vi "SecondsToHMS.vi"() -> ()   [LabVIEW 2014]
panel:
  out "Seconds":dbl
  out "Minutes":dbl
  out "Hours":dbl
  in  "Total Time in Seconds":dbl
  # "Converts time in seconds to hours, minutes and seconds"
  # "Control"
  # "Indicator"
  # "Indicator"
  # "Indicator"
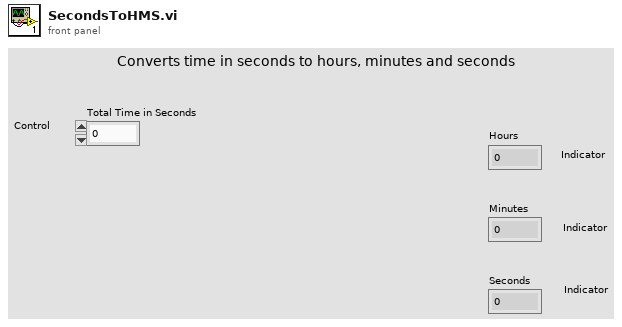
[diagram p1: front panel]
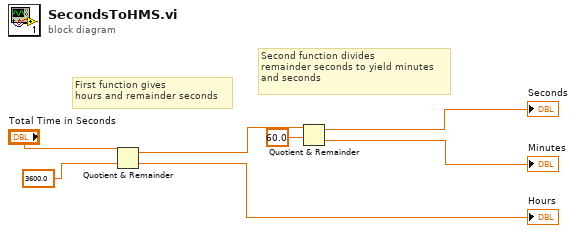
[diagram p0: block diagram]
diagram:
  # "Second function divides\nremainder seconds to yield minutes\nand seconds"
  # "First function gives\nhours and remainder seconds"
  n1 = Quotient & Remainder(x="Total Time in Seconds", y=3600.0) -> (x-y*floor(x/y)=w4:dbl, floor(x/y)=→"Hours":dbl)
  n2 = Quotient & Remainder(x=w4, y=60.0) -> (x-y*floor(x/y)=→"Seconds":dbl, floor(x/y)=→"Minutes":dbl)
